vi "Counts Update (manual).vi"(5 "Perf":T1, 6 "output cluster":T3, 7 "Cluster":cluster{"Time":timestamp, "Auto Times":T2}, 8 "Desired Cycle Time (s)":dbl=2.0, 9 "AVL":dbl=100.0 min=0.0 max=100.0 step=0.1, 10 "OutputCount":u32, 11 "Counts in":cluster{"OutputCount":u32, "RejectCount":u32}) -> (1 "OEE":T4={"AVL"=100.0, "PRF"=100.0, "QUA"=100.0, "OEE"=0.0} {"OEE" format="%#.1f"; "QUA" min=0.0 max=100.0 step=0.1; "PRF" min=0.0 max=100.0 step=0.1; "AVL" min=0.0 max=100.0 step=0.1}, 3 "Counts out":cluster{"OutputCount":u32, "RejectCount":u32})   [LabVIEW 2021]
uses:
  RT/Controls/Auto Times.ctl
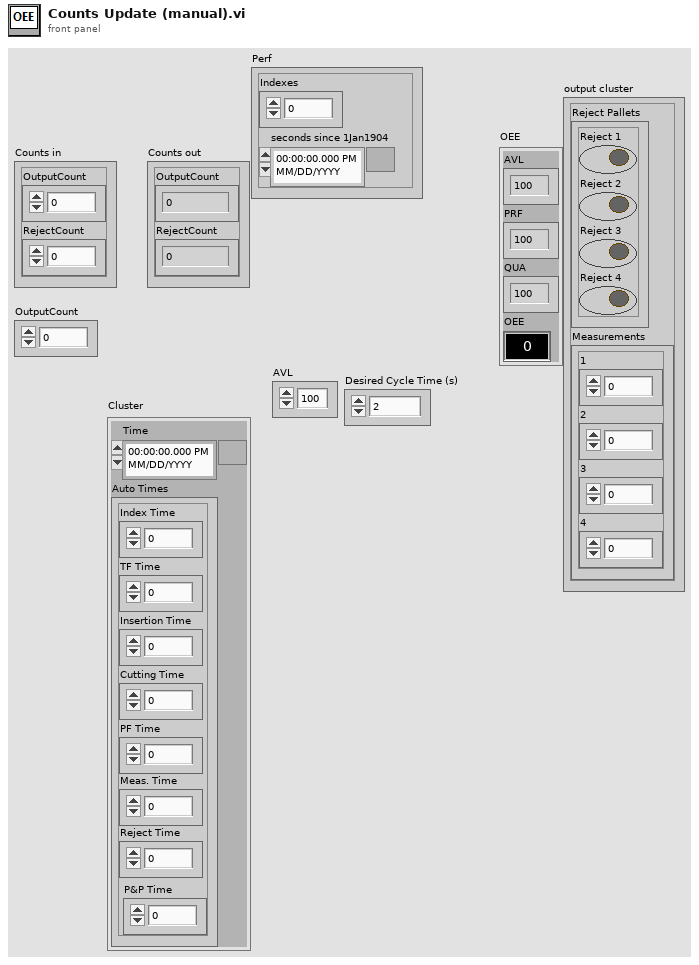
[diagram p1: front panel]
types:
  T1 = cluster{"Indexes":i32, "seconds since 1Jan1904":timestamp}
  T2 = typedef "Auto Times.ctl" = cluster{"Index Time":u32, "TF Time":u32, "Insertion Time":u32, "Cutting Time":u32, "PF Time":u32, "Meas. Time":u32, "Reject Time":u32, "P&P Time":u32}
  T3 = cluster{"Reject Pallets":cluster{"Reject 1":bool, "Reject 2":bool, "Reject 3":bool, "Reject 4":bool}, "Measurements":cluster{"1":dbl, "2":dbl, "3":dbl, "4":dbl}}
  T4 = cluster{"AVL":dbl, "PRF":dbl, "QUA":dbl, "OEE":dbl}
  T5 = cluster{"Reject 1":bool, "Reject 2":bool, "Reject 3":bool, "Reject 4":bool}
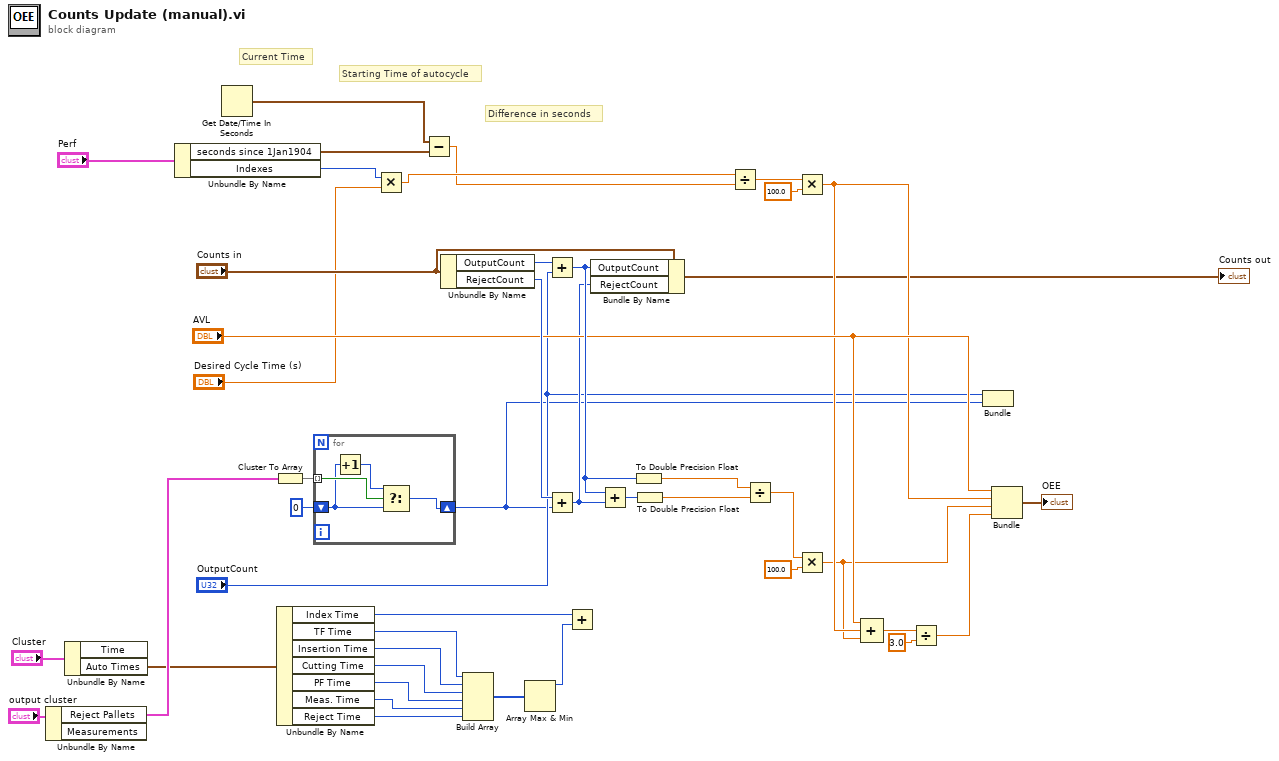
[diagram p0: block diagram]
diagram:
  # "Difference in seconds"
  # "Starting Time of autocycle"
  # "Current Time"
  n1 = Unbundle By Name("output cluster") -> ("Reject Pallets"=w10:T5)  [unwired: 1 out]
  n2 = Unbundle By Name("Cluster") -> ("Auto Times"=w8:T2)  [unwired: 1 out]
  n3 = Unbundle By Name("Perf") -> ("seconds since 1Jan1904"=w5:timestamp, "Indexes"=w3:i32)
  n4 = Get Date/Time In Seconds() -> (seconds since 1Jan1904=w6:timestamp)
  n5 = Cluster To Array(cluster=w10) -> (array=w42:bool[])
  n6 = Unbundle By Name(w8) -> ("Index Time"=w33:u32, "TF Time"=w27:u32, "Insertion Time"=w28:u32, "Cutting Time"=w29:u32, "PF Time"=w30:u32, "Meas. Time"=w31:u32, "Reject Time"=w32:u32)
  n7 = for {
    tunnel: w42 -> [w48] mode=indexing
    shift-right: [w47] -> w14
    shift-left: u32 0 -> [w46]
    n8 = Increment(x=w46) -> (x+1=w45:u32)
    n9 = Select(t=w45, s=w48, f=w46) -> (s? t:f=w47:u32)
  }
  n10 = Multiply(x=w3, y="Desired Cycle Time (s)") -> (x*y=w2:dbl)
  n11 = Subtract(x=w6, y=w5) -> (x-y=w1:dbl)
  n12 = Unbundle By Name("Counts in") -> ("OutputCount"=w44:u32, "RejectCount"=w43:u32)
  n13 = Build Array(w27, w28, w29, w30, w31, w32) -> (w26:u32[])
  n14 = Array Max & Min(array=w26) -> (max value=w25:u32)  [unwired: 3 out]
  n15 = Add(x=w44, y="OutputCount") -> (x+y=w38:u32)
  n16 = Add(x=w43, y=w14) -> (x+y=w16:u32)
  n17 = Add(x=w33, y=w25) -> ()  [unwired: 1 out]
  n18 = Bundle By Name(cluster="Counts in", "OutputCount"=w38, "RejectCount"=w16) -> (→"Counts out":cluster{"OutputCount":u32, "RejectCount":u32})
  n19 = Add(x=w38, y=w16) -> (x+y=w39:u32)
  n20 = To Double Precision Float(number=w38) -> (double precision float=w18:dbl)
  n21 = To Double Precision Float(number=w39) -> (double precision float=w17:dbl)
  n22 = Divide(x=w2, y=w1) -> (x/y=w23:dbl)
  n23 = Divide(x=w18, y=w17) -> (x/y=w36:dbl)
  n24 = Multiply(x=w23, y=100.0) -> (x*y=w20:dbl)
  n25 = Multiply(x=w36, y=100.0) -> (x*y=w19:dbl)
  n26 = Compound Arithmetic op=ADD("AVL", w20, w19) -> (w37:dbl)
  n27 = Divide(x=w37, y=3.0) -> (x/y=w21:dbl)
  n28 = Bundle("OutputCount"="OutputCount", w14) -> ()  [unwired: 1 in, 1 out]
  n29 = Bundle("AVL"="AVL", w20, w19, w21) -> (→"OEE":cluster{"AVL":dbl, dbl, dbl, dbl})  [unwired: 1 in]
